vi "Update ROI.vi"(8 "error in (no error)":errorcluster, 11 "Detail Graph in":refnum<class "Detail Graph.lvclass">) -> (0 "error out":errorcluster, 3 "Detail Graph out":refnum<class "Detail Graph.lvclass">)   [LabVIEW 2023, in "Detail Graph.lvclass"]
uses:
  Detail Graph.lvclass
  Detail Graph.lvclass/Detail Graph.ctl
  Base Graph/Base Graph.lvclass
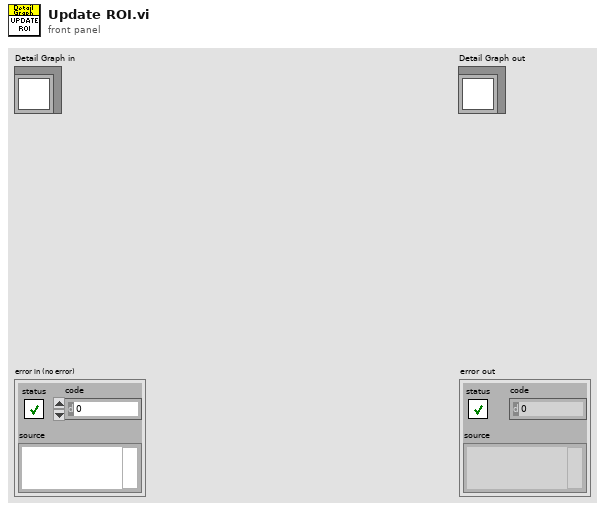
[diagram p1: front panel]
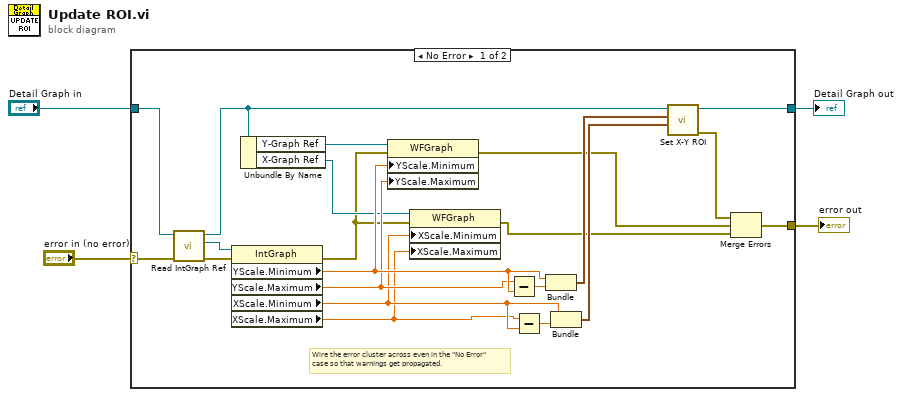
[diagram p0: block diagram]
diagram:
  n1 = case shown="No Error" "error in (no error)" {
    selector: "error in (no error)" -> [w24 w27]
    tunnel: [w7 w27] -> w3
    tunnel: [w21 w26] -> w1
    tunnel: "Detail Graph in" -> [w25 w26]
    frame No Error {
      # "Wire the error cluster across even in the \"No Error\"\ncase so that warnings get propagated."
      n2 = call "Read IntGraph Ref.vi"("error in (no error)"=w24, "TG Base Graph in"=w25) -> ("error out"=w22:errorcluster, "IntGraph Ref"=w23:refnum<vi>, "TG Base Graph out"=w15:refnum<class "Detail Graph.lvclass">)  [unwired: 7 in]
      n3 = property on="Property Node" class="IntGraph"(reference=w23, error in=w22) -> (error out=w10:errorcluster, "YScale.Minimum"=w13:dbl, "YScale.Maximum"=w12:dbl, "XScale.Minimum"=w9:dbl, "XScale.Maximum"=w8:dbl)  [unwired: 1 out]
      n4 = Unbundle By Name(w15) -> ("Y-Graph Ref"=w14:refnum<vi>, "X-Graph Ref"=w11:refnum<vi>)
      n5 = property on="Property Node" class="WFGraph"(reference=w14, error in=w10, "YScale.Minimum"=w13, "YScale.Maximum"=w12) -> (error out=w6:errorcluster)  [unwired: 1 out]
      n6 = property on="Property Node" class="WFGraph"(reference=w11, error in=w10, "XScale.Minimum"=w9, "XScale.Maximum"=w8) -> (error out=w5:errorcluster)  [unwired: 1 out]
      n7 = Subtract(x=w12, y=w13) -> (x-y=w18:dbl)
      n8 = Subtract(x=w8, y=w9) -> (x-y=w20:dbl)
      n9 = Bundle("YScale.Minimum"=w13, w18) -> (w17:cluster{"YScale.Minimum":dbl, dbl})  [unwired: 1 in]
      n10 = Bundle("XScale.Minimum"=w9, w20) -> (w19:cluster{"XScale.Minimum":dbl, dbl})  [unwired: 1 in]
      n11 = call-dynamic "Set X-Y ROI.vi"("ROI X"=w19, "ROI Y"=w17, "TG Base Graph in"=w15) -> ("error out"=w16:errorcluster, "TG Base Graph out"=w21:refnum<class "Detail Graph.lvclass">)  [unwired: 7 in]
      n12 = Merge Errors(w16, w6, w5) -> (w7:errorcluster)
    }
    frame Error {
    }
  }
  "error out" <- w3
  "Detail Graph out" <- w1
